vi "WriteConfiguration_VI.vi"(8 "error in":errorcluster, 11 "PythonConverter_GUI in":refnum<class "PythonConverter_GUI.lvclass">) -> (0 "error out":errorcluster, 3 "PythonConverter_GUI out":refnum<class "PythonConverter_GUI.lvclass">)   [LabVIEW 2014, in "Raspberry Pi Compatible Compiler for LabVIEW.lvlib" / "PythonConverter_GUI.lvclass"]
uses:
  PythonConverter_GUI.lvclass
  PythonConverter_GUI.lvclass/PythonConverter_GUI.ctl
  PythonConfiguration/PythonConfiguration.lvclass/PythonConfiguration.ctl
  VI Interpreter/Classes/VI Interpreter/VI Interpreter.lvclass/VI Interpreter.ctl
  VI Interpreter/Classes/VI Interpreter/VI Interpreter.lvclass
  PythonConfiguration/PythonConfiguration.lvclass
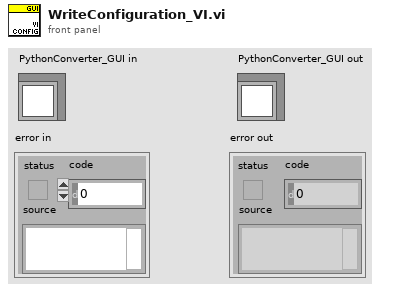
[diagram p1: front panel]
types:
  T1 = typedef "Raspberry Pi Compatible Compiler for LabVIEW.lvlib/PythonConfiguration.lvclass/ItemTD.ctl" = cluster{"Key":string, "Value":string}
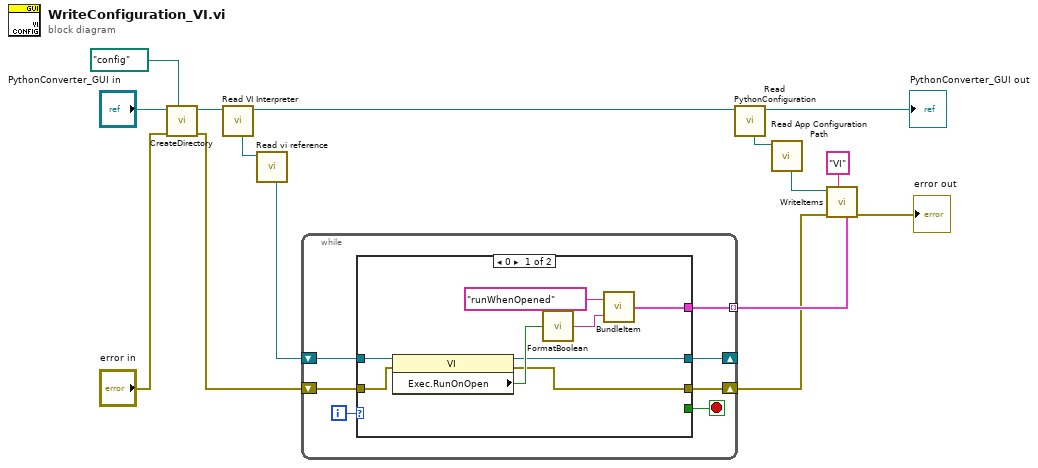
[diagram p0: block diagram]
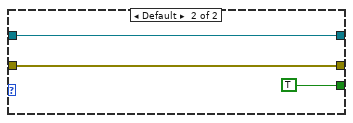
[diagram p2: hidden frame]
diagram:
  n1 = call "CreateDirectory.vi"("Relative Path"=path "config", "error in"="error in", "PythonConverter_GUI in"="PythonConverter_GUI in") -> ("error out"=w3:errorcluster, "PythonConverter_GUI out"=w5:refnum<class "PythonConverter_GUI.lvclass">)  [unwired: 4 in, 1 out]
  n2 = call "Read VI Interpreter.vi"("PythonConverter_GUI in"=w5) -> ("PythonConverter_GUI out"=w1:refnum<class "PythonConverter_GUI.lvclass">, "VI Interpreter"=w9:refnum<class "VI Interpreter.lvclass">)  [unwired: 7 in]
  n3 = call "Read vi reference.vi"("VI Interpreter in"=w9) -> ("vi reference"=w8:refnum<vi>)  [unwired: 7 in, 1 out]
  n4 = while {
    shift-right: [w20] -> _
    shift-left: w8 -> [w21]
    tunnel: [w19] -> w13 mode=indexing
    shift-right: [w16] -> w7
    shift-left: w3 -> [w17]
    i -> [w22]
    stop <- w18 stop-if-true
    n5 = case shown="0" w22 {
      tunnel: w21 -> [w24 w33]
      tunnel: [w26 w33] -> w20
      tunnel: [w28 _] -> w19
      tunnel: [_ TRUE] -> w18
      tunnel: w17 -> [w25 w31]
      tunnel: [w23 w31] -> w16
      frame 0 {
        n6 = property class="VI"(reference=w24, error in=w25) -> (reference out=w26:refnum<vi>, error out=w23:errorcluster, "Exec.RunOnOpen"=w27:bool)
        n7 = call "FormatBoolean.vi"("boolean"=w27) -> ("value"=w29:string)
        n8 = call "BundleItem.vi"("Value"=w29, "Key"="runWhenOpened") -> ("Item"=w28:T1)
      }
      frame Default {
      }
    }
  }
  n9 = call "Read PythonConfiguration.vi"("PythonConverter_GUI in"=w1) -> ("PythonConverter_GUI out"=→"PythonConverter_GUI out":refnum<class "PythonConverter_GUI.lvclass">, "PythonConfiguration"=w14:refnum<class "PythonConfiguration.lvclass">)  [unwired: 7 in]
  n10 = call "Read App Configuration Path.vi"("PythonConfiguration in"=w14) -> ("App Configuration Path"=w15:path)  [unwired: 7 in, 1 out]
  n11 = call "WriteItems.vi"("Items"=w13, "section"="VI", "error in"=w7, "Path"=w15) -> ("error out"=→"error out":errorcluster)  [unwired: 5 in]
